vi "FGV Graphen Daten.vi"(11 "error in (no error)":errorcluster caption="Fehler (Eingang, kein Fehler)", 13 "Aktion":T1) -> (4 "Waveform":waveform(sgl), 8 "Istwert":sgl, 15 "error out":errorcluster caption="Fehler (Ausgang)")   [LabVIEW 2020, in "EPA 1065.lvlib" / "ARN Test 1065-305.lvlib"]
uses:
  ARN Test 1065-305.lvlib
  Aktion FGV Graphen Daten.ctl
  Aktion FGV ARN Daten.ctl
  Messdaten/Aktionen FGV Messdaten.ctl
  Messdaten/Messdaten.lvlib
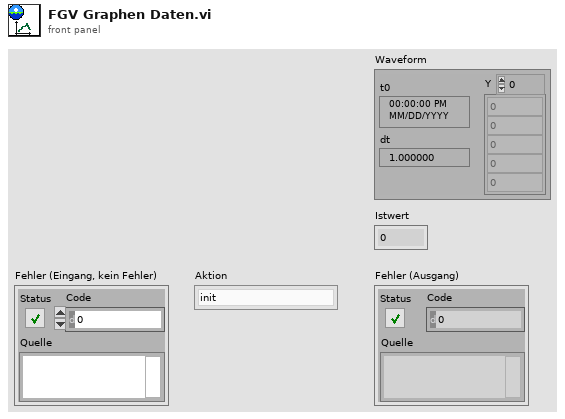
[diagram p1: front panel]
types:
  T1 = typedef "EPA 1065.lvlib/ARN Test 1065-305.lvlib/Aktion FGV Graphen Daten.ctl" = enum16{"init", "lesen", "Daten schreiben"}
  T2 = enum16{"init", "lesen", "ARN Test aktiv", "ARN Test inaktiv"}
  T3 = typedef "EPA 1065.lvlib/ARN Test 1065-305.lvlib/Aktion FGV ARN Daten.ctl" = enum16{"Lesen", "laden", "speichern", "ARN Daten", "Rohdaten", "Rohdaten löschen", "Zeitstempel", "SNR Ergebnis"}
  T4 = typedef "Messdaten.lvlib/Aktionen FGV Messdaten.ctl" = enum16{"lesen", "schreiben", "löschen", "Mittelwerte", "Komponente"}
  T5 = typedef "EPA 1065.lvlib/ARN Test 1065-305.lvlib/Allgemeine Einstellungen.ctl" = cluster{"Bearbeiter:":string, "Analysator":T6, "Komponente:":u16, "Gasflaschen Nr.:":string, "Accuracy":dbl, "Sollwert":dbl, "Modus":T7, "Pfad:":path, "Textname:":string, "CG Aufschaltzeit:":dbl, "Einheit":string, "N2 Aufschaltzeit:":dbl, "Gasflasche":T8, "Konfig Gasflasche":T9}
  T6 = typedef "System Einstellungen V2.lvlib/Analysatoren.ctl" = string
  T7 = typedef "EPA 1065.lvlib/T90 Test 1065-308.lvlib/Modus.ctl" = u16
  T8 = typedef "System Einstellungen V2.lvlib/Gasflasche Auswahl.ctl" = u16
  T9 = typedef "System Einstellungen V2.lvlib/Konfig Gasflasche.ctl" = bool
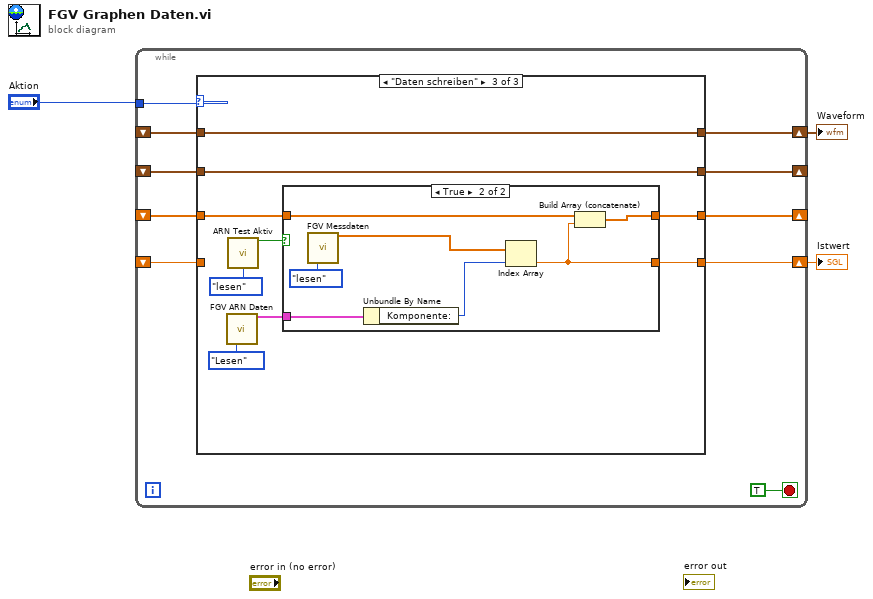
[diagram p0: block diagram]
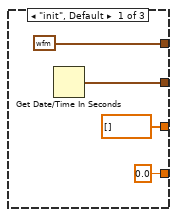
[diagram p2: hidden frame]
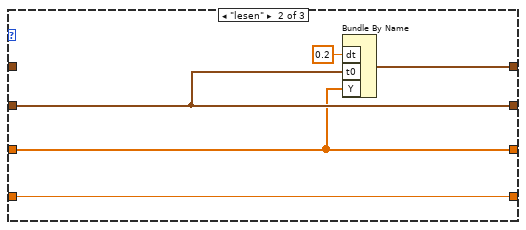
[diagram p3: hidden frame]
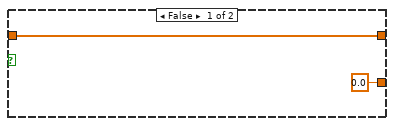
[diagram p4: hidden frame]
diagram:
  n1 = while {
    tunnel: "Aktion" -> [w13]
    shift-right: [w11] -> _
    shift-left: _ -> [w10]
    shift-right: [w9] -> _
    shift-left: _ -> [w8]
    shift-right: [w7] -> w1
    shift-left: _ -> [w6]
    shift-right: [w5] -> w2
    shift-left: _ -> [w4]
    stop <- TRUE stop-if-true
    n2 = case shown="\"Daten schreiben\"" w13 {
      tunnel: [sgl[] [] w19 w31] -> w11
      tunnel: w10 -> [_ w19 w30]
      tunnel: [w17 w20 w29] -> w9
      tunnel: w8 -> [_ w20 w29]
      tunnel: [sgl 0.0 ("Numerisch") w21 w28] -> w7
      tunnel: w6 -> [_ w21 _]
      tunnel: [waveform(sgl) {"t0"=timestamp(0 s since 1904-01-01), "dt"=1.0, "Y"=[]} w18 w25] -> w5
      tunnel: w4 -> [_ _ w25]
      frame "init", Default {
        n3 = Get Date/Time In Seconds() -> (seconds since 1Jan1904=w17:timestamp)
      }
      frame "lesen" {
        n4 = Bundle By Name("dt"=0.2, "t0"=w20, "Y"=w19) -> (w18:waveform(sgl))  [unwired: 1 in]
      }
      frame "Daten schreiben" {
        n5 = call "FGV ARN Daten.vi"("Aktion"=Aktion_FGV_ARN_Daten."Lesen") -> ("ARN Konfig Daten"=w27:T5)  [unwired: 9 in, 5 out]
        n6 = call "ARN Test Aktiv.vi"("Aktion"=T2."lesen") -> ("ARN Test Aktiv"=w23:bool)  [unwired: 13 in, 1 out]
        n7 = case shown="True" w23 {
          tunnel: [sgl 0.0 ("Numerisch") w38] -> w28
          tunnel: [w32 w37] -> w31
          tunnel: w30 -> [w32 w36]
          tunnel: w27 -> [_ w35]
          frame False {
          }
          frame True {
            n8 = call "FGV Messdaten.vi"("Aktionen"=Aktionen_FGV_Messdaten."lesen") -> ("Aktuelle Messwerte"=w39:sgl[])  [unwired: 6 in, 8 out]
            n9 = Unbundle By Name(w35) -> ("Komponente:"=w34:u16)
            n10 = Index Array(array=w39, index=w34) -> (element=w38:sgl)
            n11 = Build Array (concatenate)(w36, w38) -> (w37:sgl[])
          }
        }
      }
    }
  }
  "Waveform" <- w2
  "Istwert" <- w1
